vi "CommonVIs_UpdateAttributesFromPropertyMethods.vi"(10 "Methods":T4[](array[typedef]), 11 "Attributes in":T1[](array[typedef])) -> (3 "Attributes out":T1[](array[typedef]))   [LabVIEW 2020]
uses:
  String/GDSString_MethodDescriptionType.ctl
  CommonVIs_AttributeType.ctl
  CommonVIs_AttributeDataType.ctl
  String/GDSString_AccessScopeModifierType.ctl
  String/GDSString_ModifierType.ctl
  CommonVIs_PropertyType.ctl
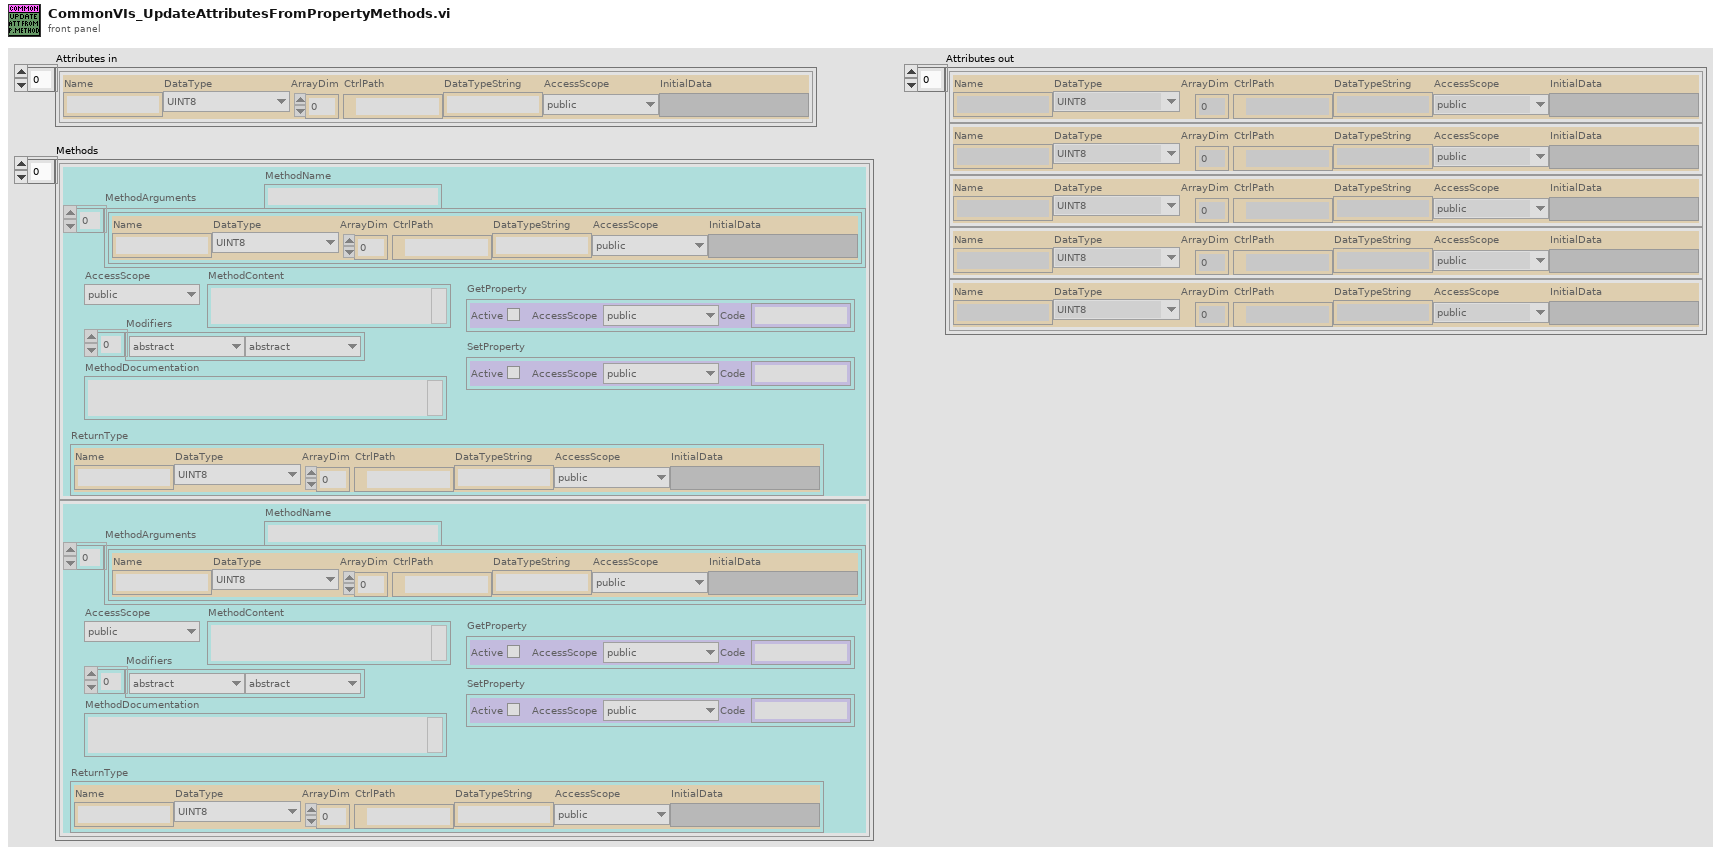
[diagram p1: front panel]
types:
  T1 = typedef "CommonVIs_AttributeType.ctl" = cluster{"Name":string, "DataType":T2, "ArrayDim":i32, "CtrlPath":path, "DataTypeString":string, "AccessScope":T3, "InitialData":variant}
  T2 = typedef "CommonVIs_AttributeDataType.ctl" = enum16{"UINT8", "INT8", "UINT16", "INT16", "UINT32", "INT32", "UINT64", "INT64", "SGL", "DBL", "EXT", "CSG", "CDB", "CXT", "TimeStamp", "STRING", "PATH", "BOOL", "ENUM", "RefNum", "VIRefNum", "LabVIEW Class", "Cluster", "Variant", "TypeDef", "Waveform", "LabVIEW Object", "Other", "void", "Set", "Map"}
  T3 = typedef "GDSString_AccessScopeModifierType.ctl" = enum16{"public", "private", "protected", "internal"}
  T4 = typedef "GDSString_MethodDescriptionType.ctl" = cluster{"ReturnType":T1, "MethodName":string, "AccessScope":T3, "Modifiers":T5[], "MethodDocumentation":string, "MethodContent":string, "MethodArguments":T1[], "GetProperty":T6, "SetProperty":T6}
  T5 = typedef "GDSString_ModifierType.ctl" = enum16{"abstract", "static", "final", "synchronized", "strictfp", "async", "const", "event", "extern", "new", "native ", "override", "partial", "readonly", "sealed", "unsafe", "virtual", "volatile"}
  T6 = typedef "CommonVIs_PropertyType.ctl" = cluster{"Active":bool, "AccessScope":T3, "Code":string}
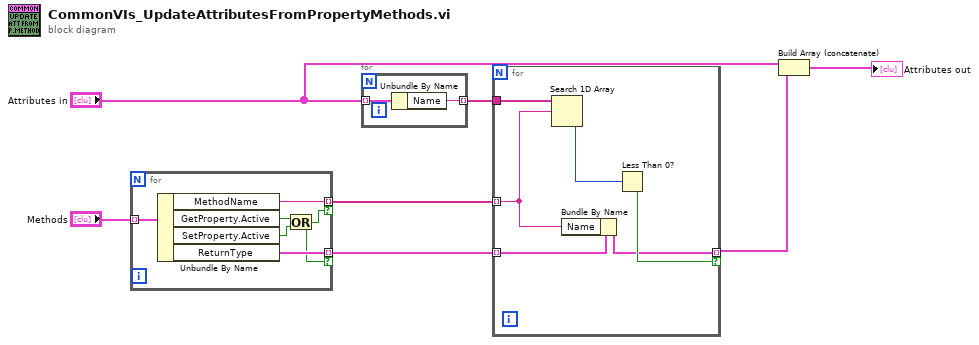
[diagram p0: block diagram]
diagram:
  n1 = for {
    tunnel: "Methods" -> [w13] mode=indexing
    tunnel: [w10] -> w5 mode=indexing if=w8
    tunnel: [w9] -> w4 mode=indexing if=w8
    n2 = Unbundle By Name(w13) -> ("MethodName"=w10:string, "GetProperty.Active"=w12:bool, "SetProperty.Active"=w11:bool, "ReturnType"=w9:T1)
    n3 = Or(x=w12, y=w11) -> (x .or. y?=w8:bool)
  }
  n4 = for {
    tunnel: "Attributes in" -> [w15] mode=indexing
    tunnel: [w14] -> w6 mode=indexing
    n5 = Unbundle By Name(w15) -> ("Name"=w14:string)
  }
  n6 = for {
    tunnel: w6 -> [w21]
    tunnel: w5 -> [w16] mode=indexing
    tunnel: w4 -> [w18] mode=indexing
    tunnel: [w17] -> w2 mode=indexing if=w19
    n7 = Search 1D Array(1D array=w21, element=w16) -> (index of element=w20:i32)  [unwired: 1 in]
    n8 = Bundle By Name(cluster=w18, "Name"=w16) -> (w17:T1)
    n9 = Less Than 0?(x=w20) -> (x < 0?=w19:bool)
  }
  n10 = Build Array (concatenate)("Attributes in", w2) -> (→"Attributes out":T1[])
